vi "Get array of DBL.vi"(8 "error in (no error)":errorcluster, 11 "json class in":refnum<class "json class.lvclass">) -> (0 "error out":errorcluster, 2 "DBL Array":dbl[](array[numeric]), 3 "json class out":refnum<class "json class.lvclass">)   [LabVIEW 2021, in "Config Library.lvlib" / "json class.lvclass"]
uses:
  json class.lvclass
  json class.lvclass/json class.ctl
  <vilib>/addons/JSON API/JSON Array/JSON Array.lvclass
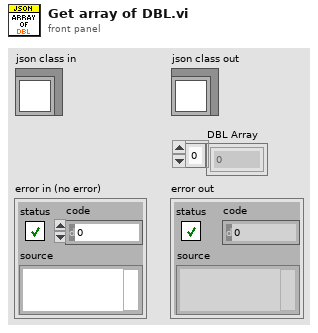
[diagram p1: front panel]
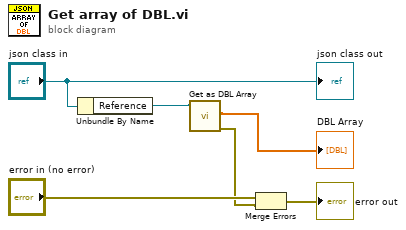
[diagram p0: block diagram]
diagram:
  n1 = Unbundle By Name("json class in") -> ("Reference"=w3:refnum<class "JSON Value.lvclass">)
  n2 = call <vilib>:"Get as DBL Array.vi"("JSON Array in"=w3) -> ("error out"=w1:errorcluster, "Array of numbers"=→"DBL Array":dbl[])  [unwired: 8 in, 1 out]
  n3 = Merge Errors("error in (no error)", w1) -> (→"error out":errorcluster)
  "json class out" <- "json class in"
